vi "Start.vi"(0 "reference in":refnum<class "Dec.lvclass">, 5 "error in (no error)":errorcluster) -> (14 "reference out":refnum<class "Dec.lvclass">, 19 "error out":errorcluster)   [LabVIEW 2013, in "Dec.lvclass"]
uses:
  Dec.lvclass
  Mech_class/Mech.lvclass
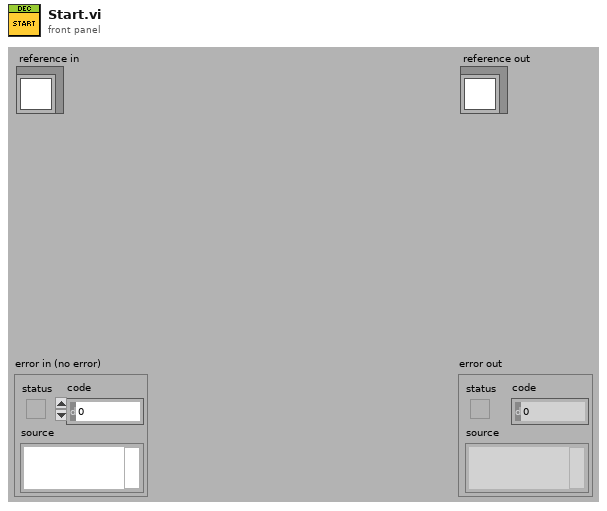
[diagram p1: front panel]
types:
  T1 = typedef "Dec.lvclass/ObjectAttributes.ctl" = cluster{"Mech.lvclass":refnum<class "Mech.lvclass">}
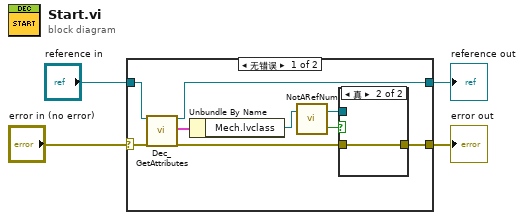
[diagram p0: block diagram]
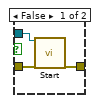
[diagram p2: hidden frame]
diagram:
  n1 = case shown="无错误" "error in (no error)" {
    selector: "error in (no error)" -> [w13 w19]
    tunnel: [w5 w19] -> w3
    tunnel: [w12 w18] -> w1
    tunnel: "reference in" -> [w10 w18]
    frame No Error {
      n2 = call "Dec_GetAttributes.vi"("reference in"=w10, "error in (no error)"=w13) -> ("reference out"=w12:refnum<class "Dec.lvclass">, "attributes"=w11:T1, "error out"=w6:errorcluster)  [unwired: 14 in, 1 out]
      n3 = Unbundle By Name(w11) -> ("Mech.lvclass"=w9:refnum<class "Mech.lvclass">)
      n4 = call-dynamic "NotARefNum.vi"("reference in"=w9) -> ("not a refnum?"=w8:bool, "reference out"=w7:refnum<class "Mech.lvclass">)  [unwired: 1 in]
      n5 = case shown="真" w8 {
        tunnel: w7 -> [w16 _]
        tunnel: w6 -> [w15 w17]
        tunnel: [w14 w17] -> w5
        frame False {
          n6 = call-dynamic "Start.vi"("reference in"=w16, "error in (no error)"=w15) -> ("error out"=w14:errorcluster)  [unwired: 16 in, 1 out]
        }
        frame True {
        }
      }
    }
    frame Error {
    }
  }
  "error out" <- w3
  "reference out" <- w1
